vi "PassFailTest.vi"(1 "[A/Ds]":dbl[][](array[numeric]), 3 "[LiveLoad]":dbl[](array[numeric]), 11 "Zero G.load":dbl) -> (4 "Pass?":bool, 6 "ScaleFactorA":u8, 8 "ScaleFactorB":u8, 10 "Pass/Fail #":i32, 14 "Test Results":dbl[][](array[numeric]) format="%.2f", 15 "May Pass Retest?":bool)   [LabVIEW 2013]
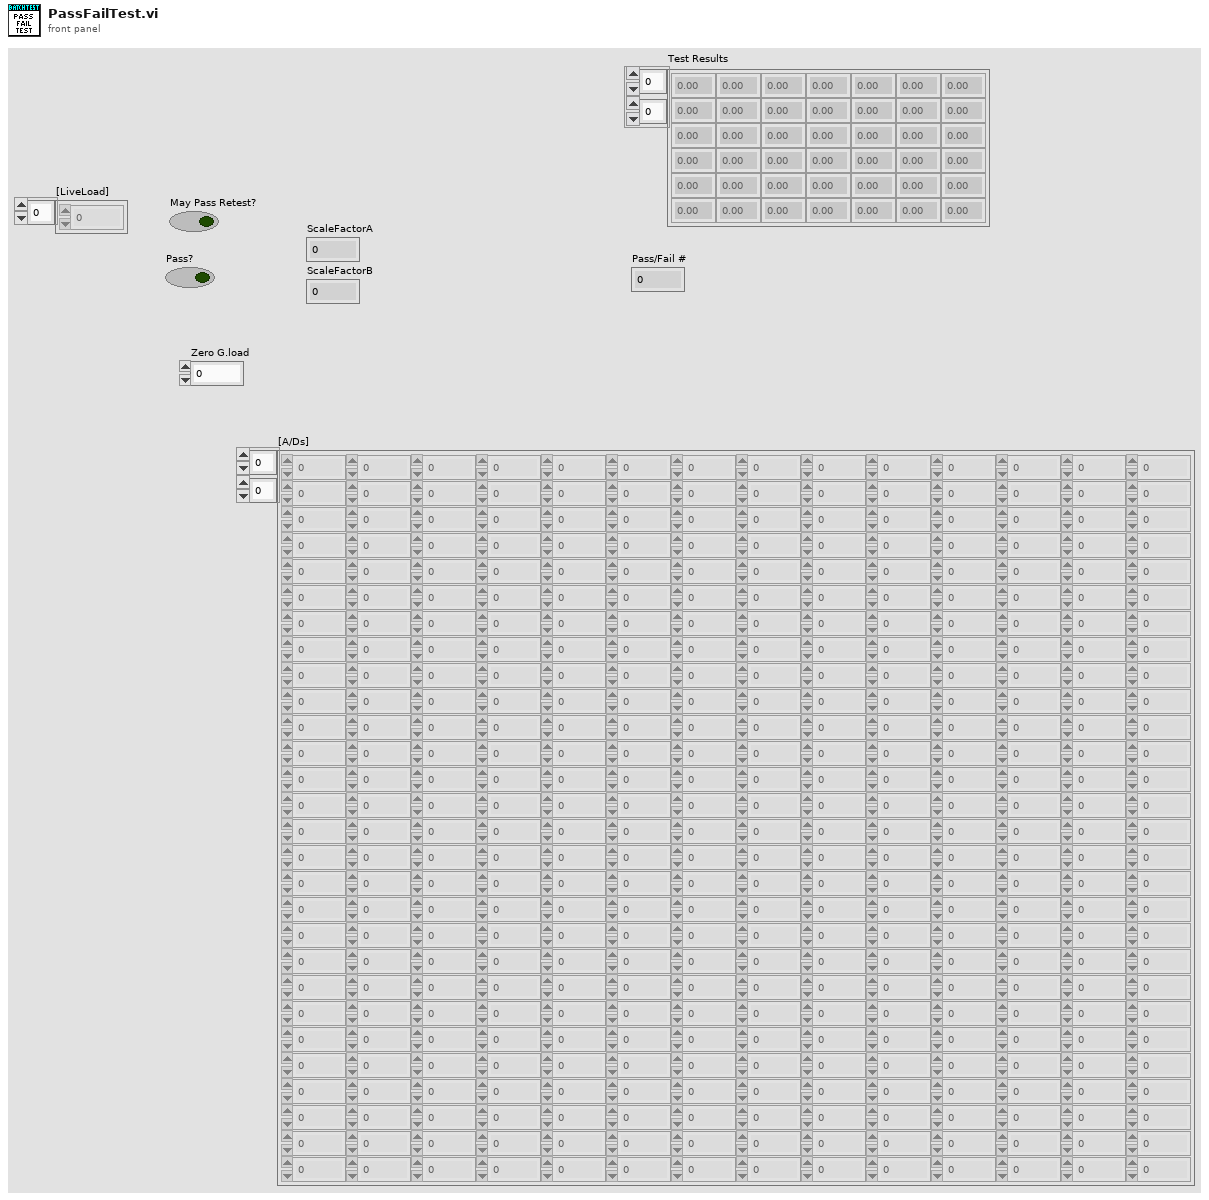
[diagram p1: front panel]
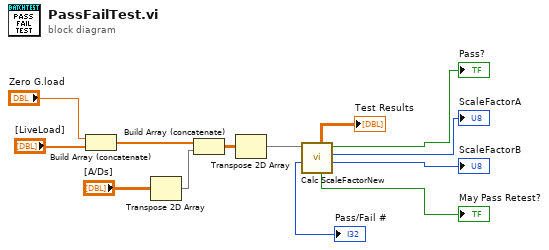
[diagram p0: block diagram]
diagram:
  n1 = Build Array (concatenate)("Zero G.load", "[LiveLoad]") -> (w8:dbl[])
  n2 = Transpose 2D Array(2D array="[A/Ds]") -> (transposed array=w4:dbl[][])
  n3 = Build Array (concatenate)(w8, w4) -> (w5:dbl[][])
  n4 = Transpose 2D Array(2D array=w5) -> (transposed array=w3:dbl[][])
  n5 = call "Calc ScaleFactorNew.vi"("[A/D Input]"=w3) -> ("ScaleFactorB"=→"ScaleFactorB":i32, "ScaleFactorA"=→"ScaleFactorA":i32, "Pass?"=→"Pass?":bool, "May Pass Retest?"=→"May Pass Retest?":bool, "Test Results"=→"Test Results":dbl[][], "Pass/Fail #"=→"Pass/Fail #":i32)  [unwired: 4 in, 1 out]
